vi "Workspace.Close.vi"(8 "Password":string, 9 "Username":string, 10 "Project File Path":path, 11 "Gateway IP Address (\"\": localhost)":string) -> (0 "error out":errorcluster)   [LabVIEW 2013, in "MiscHelperVIs.lvlib"]
uses:
  MiscHelperVIs.lvlib
  <vilib>/NI Veristand/Execution/Project/NI_VS Project ExecutionAPI.lvlib
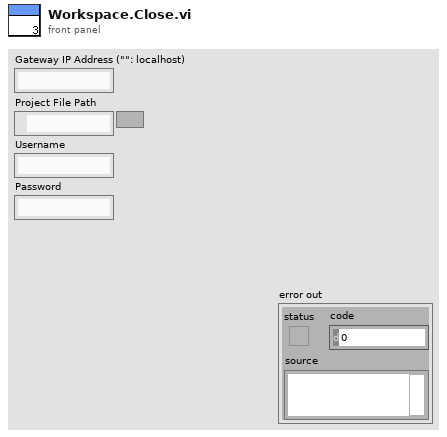
[diagram p1: front panel]
types:
  T1 = typedef "NI_VS Project ExecutionAPI.lvlib/Project Ref.ctl" = refnum<k24>
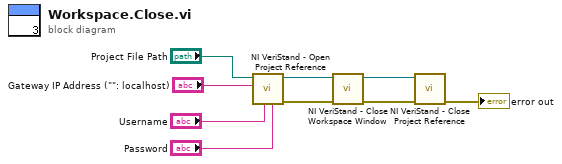
[diagram p0: block diagram]
diagram:
  n1 = call <vilib>:"NI VeriStand - Open Project Reference.vi"("Password"="Password", "Username"="Username", "Gateway IP Address (\"\": localhost)"="Gateway IP Address (\"\": localhost)", "Project File Path"="Project File Path") -> ("error out"=w9:errorcluster, "Project Ref"=w6:T1)  [unwired: 6 in]
  n2 = call <vilib>:"NI VeriStand - Close Workspace Window.vi"("error in (no error)"=w9, "Project Ref in"=w6) -> ("error out"=w8:errorcluster, "Project Ref out"=w7:T1)  [unwired: 8 in]
  n3 = call <vilib>:"NI VeriStand - Close Project Reference.vi"("error in (no error)"=w8, "Project Ref"=w7) -> ("error out"=→"error out":errorcluster)  [unwired: 9 in]
